vi "Write hostname.vi"(10 "hostname":string, 11 "address":refnum<class "Hostname Network Address.lvclass">) -> (3 "address out":refnum<class "Hostname Network Address.lvclass">)   [LabVIEW 2020, in "NI_WFCN.lvlib" / "Hostname Network Address.lvclass"]
doc: "Encapsulate a hostname string into a Hostname Network Address."
uses:
  <vilib>/net/WFCN/Addressing/Hostname Network Address/Hostname Network Address.lvclass
  <vilib>/net/WFCN/Addressing/Hostname Network Address/Hostname Network Address.lvclass/Hostname Network Address.ctl
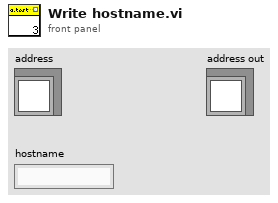
[diagram p1: front panel]
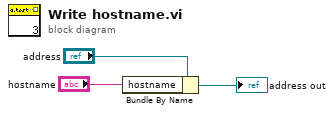
[diagram p0: block diagram]
diagram:
  n1 = Bundle By Name(cluster="address", "hostname"="hostname") -> (→"address out":refnum<class "Hostname Network Address.lvclass">)
